vi "Object Storage With Type Preservation.vi"(8 "error in (no error)":errorcluster, 10 "Action":u16(ring) items=["Store Object", "Retrieve Object"], 11 "Object in":refnum<class "Parent.lvclass">) -> (0 "error out":errorcluster, 3 "Object out":refnum<class "Parent.lvclass">)   [LabVIEW 2023, in "Parent.lvclass"]
doc: "Demonstrates different ways of store objects in shift registers, some of which will return objects using the run-time type of the Object passed in (which can include child classes of Object)."
uses:
  Parent.lvclass
panel:
  in  "Loop Count 2":i32=1
  in  "Loop Count":i32=1
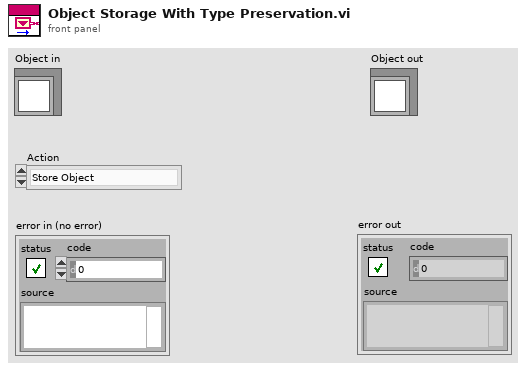
[diagram p1: front panel]
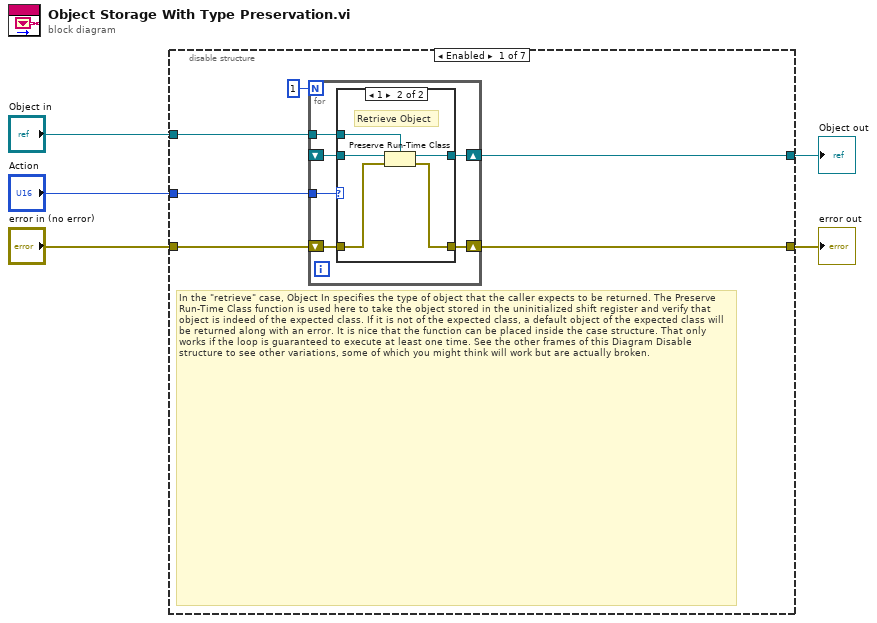
[diagram p0: block diagram]
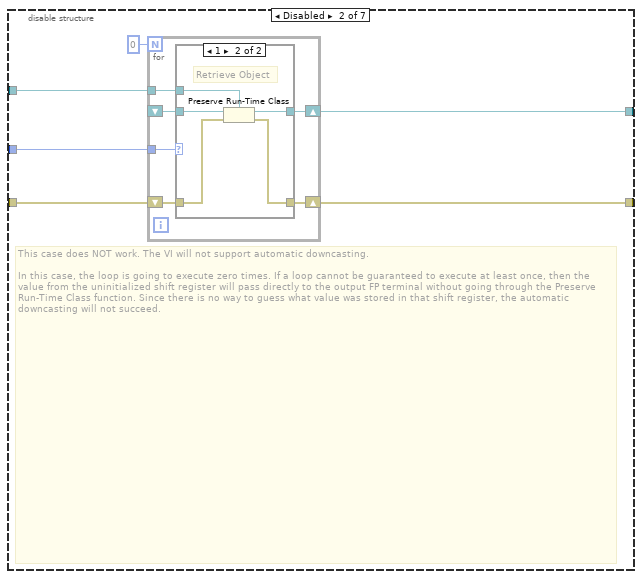
[diagram p3: hidden frame]
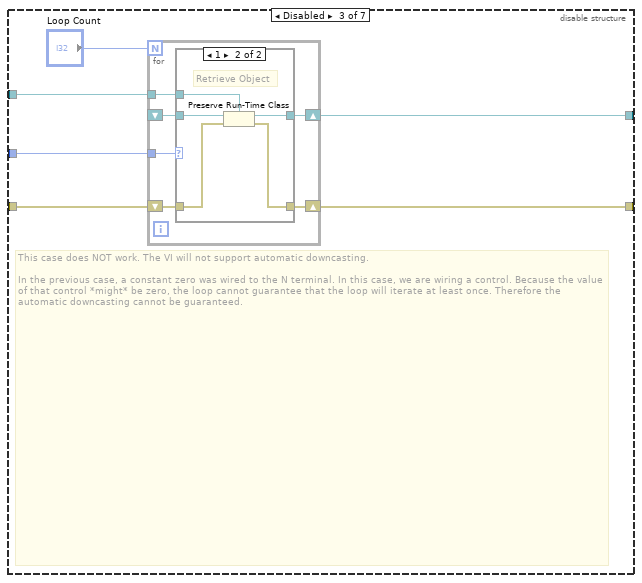
[diagram p5: hidden frame]
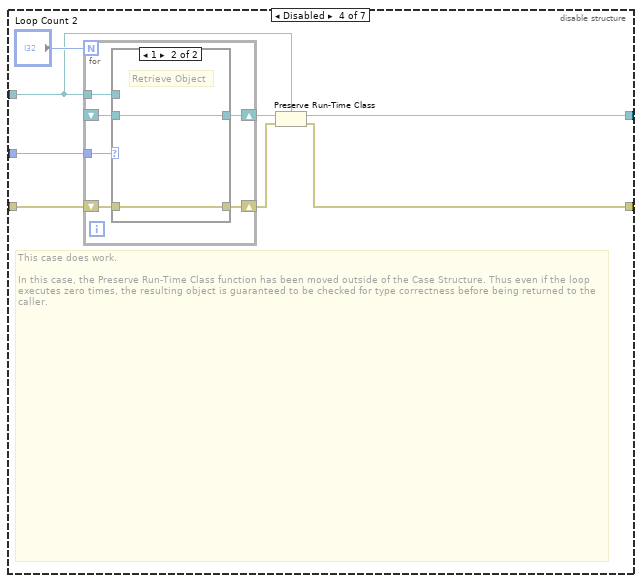
[diagram p7: hidden frame]
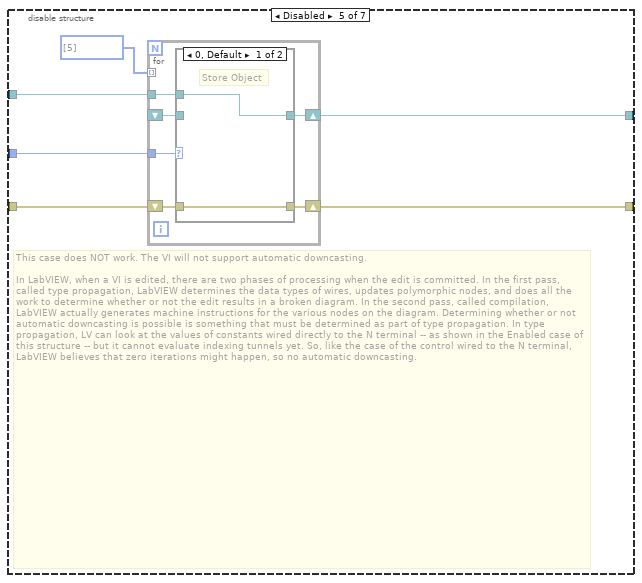
[diagram p9: hidden frame]
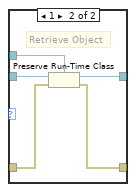
[diagram p10: hidden frame]
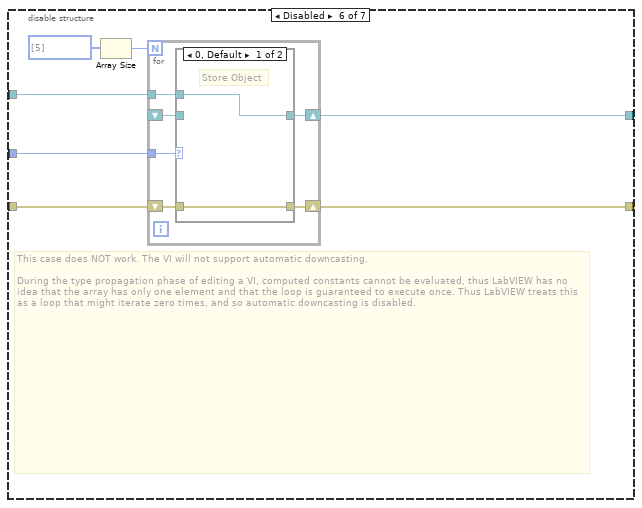
[diagram p11: hidden frame]
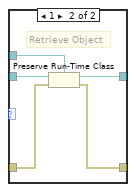
[diagram p12: hidden frame]
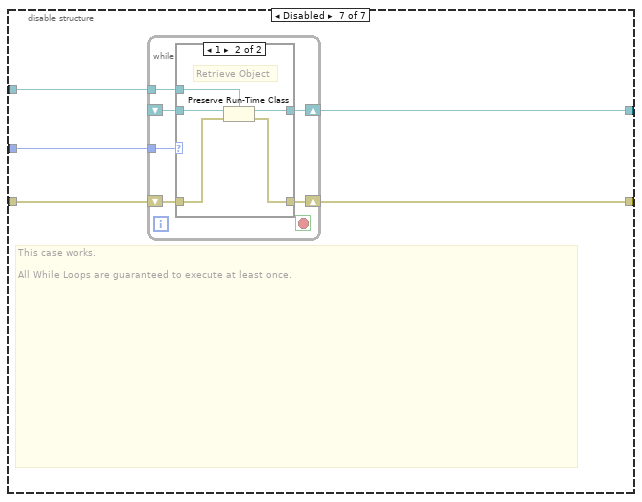
[diagram p13: hidden frame]
diagram:
  n1 = disable-structure "Diagram Disable Structure" shown="Enabled" {
    disable-tunnel: "Action" -> [w10 w29 w48 w69 w86 w106 w124]
    disable-tunnel: "Object in" -> [w9 w28 w47 w63 w85 w105 w123]
    disable-tunnel: [w8 w27 w46 w66 w84 w104 w122] -> w3
    disable-tunnel: "error in (no error)" -> [w7 w26 w45 w68 w83 w103 w121]
    disable-tunnel: [w6 w25 w44 w64 w82 w102 w120] -> w1
    frame Enabled {
      # "In the \"retrieve\" case, Object In specifies the type of object that the caller expects to be returned. The Preserve Run-Time Class function is used here to take the object stored in the uninitialized shift register and verify that object is indeed of the expected class. If it is not of the expected class, a default object of the expected class will be returned along with an error. It is nice that the function can be placed inside the case structure. That only works if the loop is guaranteed to execute at least one time. See the other frames of this Diagram Disable structure to see other variations, some of which you might think will work but are actually broken."
      n2 = for {
        N: 1 -> [_]
        shift-right: [w16] -> w8
        shift-left: _ -> [w14]
        tunnel: w10 -> [w17]
        tunnel: w9 -> [w15]
        shift-right: [w12] -> w6
        shift-left: w7 -> [w13]
        n3 = case shown="1" w17 {
          tunnel: [w19 w22] -> w16
          tunnel: w15 -> [w19 w23]
          tunnel: w14 -> [_ w24]
          tunnel: w13 -> [w18 w21]
          tunnel: [w18 w20] -> w12
          frame 0, Default {
            # "Store Object"
          }
          frame 1 {
            # "Retrieve Object"
            n4 = Preserve Run-Time Class(object in=w24, error in=w21, 2:w23) -> (object out=w22:refnum<class "Parent.lvclass">, error out=w20:errorcluster)
          }
        }
      }
    }
    frame Disabled {
      # "This case does NOT work. The VI will not support automatic downcasting.\n\nIn this case, the loop is going to execute zero times. If a loop cannot be guaranteed to execute at least once, then the value from the uninitialized shift register will pass directly to the output FP terminal without going through the Preserve Run-Time Class function. Since there is no way to guess what value was stored in that shift register, the automatic downcasting will not succeed."
      n5 = for {
        N: 0 -> [_]
        shift-right: [w35] -> w27
        shift-left: _ -> [w33]
        tunnel: w29 -> [w36]
        tunnel: w28 -> [w34]
        shift-right: [w31] -> w25
        shift-left: w26 -> [w32]
        n6 = case shown="1" w36 {
          tunnel: [w38 w41] -> w35
          tunnel: w34 -> [w38 w42]
          tunnel: w33 -> [_ w43]
          tunnel: w32 -> [w37 w40]
          tunnel: [w37 w39] -> w31
          frame 0, Default {
            # "Store Object"
          }
          frame 1 {
            # "Retrieve Object"
            n7 = Preserve Run-Time Class(object in=w43, error in=w40, 2:w42) -> (object out=w41:refnum<class "Parent.lvclass">, error out=w39:errorcluster)
          }
        }
      }
    }
    frame Disabled {
      # "This case does NOT work. The VI will not support automatic downcasting.\n\nIn the previous case, a constant zero was wired to the N terminal. In this case, we are wiring a control. Because the value of that control *might* be zero, the loop cannot guarantee that the loop will iterate at least once. Therefore the automatic downcasting cannot be guaranteed."
      n8 = for {
        N: "Loop Count" -> [_]
        shift-right: [w54] -> w46
        shift-left: _ -> [w52]
        tunnel: w48 -> [w55]
        tunnel: w47 -> [w53]
        shift-right: [w50] -> w44
        shift-left: w45 -> [w51]
        n9 = case shown="1" w55 {
          tunnel: [w57 w60] -> w54
          tunnel: w53 -> [w57 w61]
          tunnel: w52 -> [_ w62]
          tunnel: w51 -> [w56 w59]
          tunnel: [w56 w58] -> w50
          frame 0, Default {
            # "Store Object"
          }
          frame 1 {
            # "Retrieve Object"
            n10 = Preserve Run-Time Class(object in=w62, error in=w59, 2:w61) -> (object out=w60:refnum<class "Parent.lvclass">, error out=w58:errorcluster)
          }
        }
      }
    }
    frame Disabled {
      # "This case does work.\n\nIn this case, the Preserve Run-Time Class function has been moved outside of the Case Structure. Thus even if the loop executes zero times, the resulting object is guaranteed to be checked for type correctness before being returned to the caller."
      n11 = for {
        N: "Loop Count 2" -> [_]
        shift-right: [w75] -> w67
        shift-left: _ -> [w73]
        tunnel: w69 -> [w76]
        tunnel: w63 -> [w74]
        shift-right: [w71] -> w65
        shift-left: w68 -> [w72]
        n12 = case shown="1" w76 {
          tunnel: [w78 w79] -> w75
          tunnel: w74 -> [w78 _]
          tunnel: w73 -> [_ w79]
          tunnel: w72 -> [w77 w80]
          tunnel: [w77 w80] -> w71
          frame 0, Default {
            # "Store Object"
          }
          frame 1 {
            # "Retrieve Object"
          }
        }
      }
      n13 = Preserve Run-Time Class(object in=w67, error in=w65, 2:w63) -> (object out=w66:refnum<class "Parent.lvclass">, error out=w64:errorcluster)
    }
    frame Disabled {
      # "This case does NOT work. The VI will not support automatic downcasting.\n\nIn LabVIEW, when a VI is edited, there are two phases of processing when the edit is committed. In the first pass, called type propagation, LabVIEW determines the data types of wires, updates polymorphic nodes, and does all the work to determine whether or not the edit results in a broken diagram. In the second pass, called compilation, LabVIEW actually generates machine instructions for the various nodes on the diagram. Determining whether or not automatic downcasting is possible is something that must be determined as part of type propagation. In type propagation, LV can look at the values of constants wired directly to the N terminal -- as shown in the Enabled case of this structure -- but it cannot evaluate indexing tunnels yet. So, like the case of the control wired to the N terminal, LabVIEW believes that zero iterations might happen, so no automatic downcasting."
      n14 = for {
        shift-right: [w91] -> w84
        shift-left: _ -> [w89]
        tunnel: w86 -> [w92]
        tunnel: w85 -> [w90]
        shift-right: [w87] -> w82
        shift-left: w83 -> [w88]
        tunnel: i32[] [5] -> [_] mode=indexing
        n15 = case shown="0, Default" w92 {
          tunnel: [w94 w97] -> w91
          tunnel: w90 -> [w94 w98]
          tunnel: w89 -> [_ w99]
          tunnel: w88 -> [w93 w96]
          tunnel: [w93 w95] -> w87
          frame 0, Default {
            # "Store Object"
          }
          frame 1 {
            # "Retrieve Object"
            n16 = Preserve Run-Time Class(object in=w99, error in=w96, 2:w98) -> (object out=w97:refnum<class "Parent.lvclass">, error out=w95:errorcluster)
          }
        }
      }
    }
    frame Disabled {
      # "This case does NOT work. The VI will not support automatic downcasting.\n\nDuring the type propagation phase of editing a VI, computed constants cannot be evaluated, thus LabVIEW has no idea that the array has only one element and that the loop is guaranteed to execute once. Thus LabVIEW treats this as a loop that might iterate zero times, and so automatic downcasting is disabled."
      n17 = Array Size(array=i32[] [5]) -> (size(s)=w101:i32)
      n18 = for {
        N: w101 -> [_]
        shift-right: [w111] -> w104
        shift-left: _ -> [w109]
        tunnel: w106 -> [w112]
        tunnel: w105 -> [w110]
        shift-right: [w107] -> w102
        shift-left: w103 -> [w108]
        n19 = case shown="0, Default" w112 {
          tunnel: [w114 w117] -> w111
          tunnel: w110 -> [w114 w118]
          tunnel: w109 -> [_ w119]
          tunnel: w108 -> [w113 w116]
          tunnel: [w113 w115] -> w107
          frame 0, Default {
            # "Store Object"
          }
          frame 1 {
            # "Retrieve Object"
            n20 = Preserve Run-Time Class(object in=w119, error in=w116, 2:w118) -> (object out=w117:refnum<class "Parent.lvclass">, error out=w115:errorcluster)
          }
        }
      }
    }
    frame Disabled {
      # "This case works.\n\nAll While Loops are guaranteed to execute at least once."
      n21 = while {
        shift-right: [w129] -> w122
        shift-left: _ -> [w127]
        tunnel: w124 -> [w130]
        tunnel: w123 -> [w128]
        shift-right: [w125] -> w120
        shift-left: w121 -> [w126]
        stop <- _ stop-if-true
        n22 = case shown="1" w130 {
          tunnel: [w132 w135] -> w129
          tunnel: w128 -> [w132 w136]
          tunnel: w127 -> [_ w137]
          tunnel: w126 -> [w131 w134]
          tunnel: [w131 w133] -> w125
          frame 0, Default {
            # "Store Object"
          }
          frame 1 {
            # "Retrieve Object"
            n23 = Preserve Run-Time Class(object in=w137, error in=w134, 2:w136) -> (object out=w135:refnum<class "Parent.lvclass">, error out=w133:errorcluster)
          }
        }
      }
    }
  }
  "Object out" <- w3
  "error out" <- w1
